vi "2_2.vi"() -> ()   [LabVIEW 2010]
panel:
  out "Кількість невірних введень":dbl
  in  "stop":bool
  in  "OK Button":bool
  in  "Пароль:":string
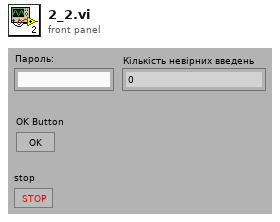
[diagram p1: front panel]
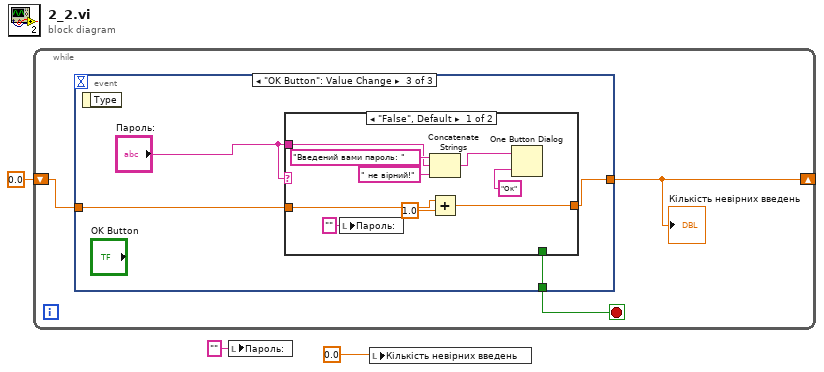
[diagram p0: block diagram]
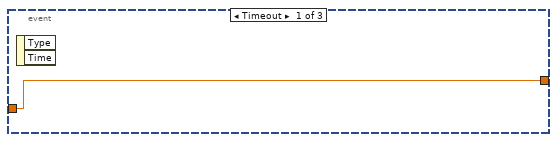
[diagram p2: hidden frame]
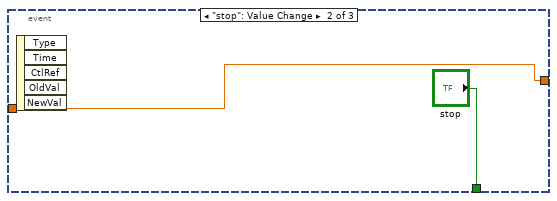
[diagram p3: hidden frame]
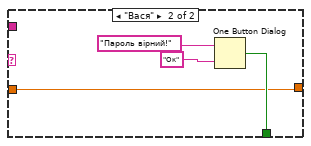
[diagram p4: hidden frame]
diagram:
  n1 = while {
    shift-right: [w4] -> _
    shift-left: 0.0 -> [w5]
    stop <- w6 stop-if-true
    n2 = event shown="[2] \"OK Button\": Value Change" {
      selector: _ -> [_ _ _]
      dyn-events: _ -> [_ _ _]
      timeout: _ -> [_ _ _]
      tunnel: [_ "stop" w13] -> w6
      tunnel: [w7 w8 w12] -> w4
      tunnel: w5 -> [w7 w8 w11]
      event Timeout {
        n3 = event-data() -> ()  [unwired: 1 in, 2 out]
      }
      event "stop": Value Change {
        n4 = event-data() -> ()  [unwired: 1 in, 5 out]
      }
      event "OK Button": Value Change {
        n5 = event-data() -> ()  [unwired: 1 in, 1 out]
        n6 = case shown="\"False\", Default" "Пароль:" {
          tunnel: [_ w24] -> w13
          tunnel: "Пароль:" -> [w20 _]
          tunnel: [w14 w23] -> w12
          tunnel: w11 -> [w16 w23]
          frame "False", Default {
            n7 = local write "Пароль:"("" ("String")) -> ()
            n8 = Concatenate Strings("Введений вами пароль: " ("string"), w20, " не вірний!" ("string")) -> (w18:string)
            n9 = Add(x=w16, y=1.0) -> (x+y=w14:dbl)
            n10 = One Button Dialog(message=w18, button name ("OK")="Ок") -> ()  [unwired: 1 out]
          }
          frame "Вася" {
            n11 = One Button Dialog(message="Пароль вірний!", button name ("OK")="Ок") -> (true=w24:bool)
          }
        }
      }
    }
    "Кількість невірних введень" <- w4
  }
  n12 = local write "Пароль:"("" ("String")) -> ()
  n13 = local write "Кількість невірних введень"(0.0 ("x+y")) -> ()
